vi "Get Part Information.vi"(8 "Error":errorcluster, 10 "station name":string, 11 "Part Type":string="WK") -> (0 "Error Out":errorcluster, 1 "Part Setup":T2={"Communication Type"=enum."None", "Send Messages to"=enum."Glass", "RAP Signal"=enum."None", "Motor Type"=enum."Smart Motor", "NVH Part Number"=0, "Turn Off Timer"=0, "Part Type"=""}, 2 "Switch Value Configuration":T7[](array[typedef]), 3 "Switch Configuration":T10[](array[typedef]), 4 "Motor Drift Compensation":i32[](array[numeric])=[25, 25, 25, 25, 25, 25, 25, 25], 5 "Seqence Info":T11[](array[typedef]), 6 "Hall Positions":i32[](array[numeric]), 7 "enable ps rem sense":bool, 9 "lvdt precision":T1)   [LabVIEW 2018]
uses:
  05.UserVI's/sequence/type defs/Sequence Info.ctl
  02.Type Def's/All Switch Configuration Cluster.ctl
  02.Type Def's/All Motions.ctl
  02.Type Def's/EOL Switch Value Configuration Cluster.ctl
  02.Type Def's/EOL Switch Max Min Check Cluster.ctl
  05.UserVI's/type defs/EOL Part Setup.ctl
  02.Type Def's/All Communication Types.ctl
  05.UserVI's/type defs/Communication with Motors.ctl
  05.UserVI's/type defs/RAP Signal Control.ctl
  05.UserVI's/type defs/EOL Motor Type.ctl
  05.UserVI's/LVDT's/lvdt precision.ctl
panel:
  # "Min"
  # "Max"
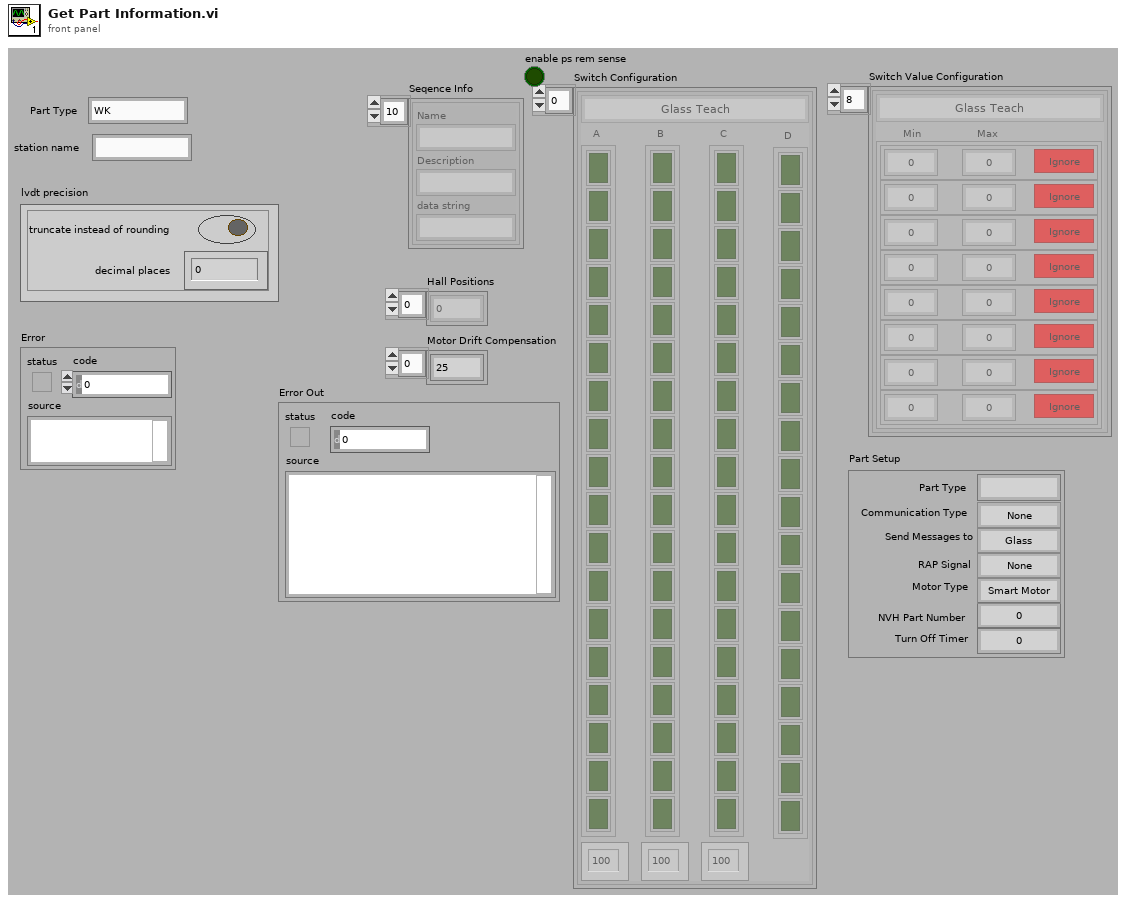
[diagram p1: front panel]
types:
  T1 = typedef "lvdt precision.ctl" = cluster{"truncate instead of rounding":bool, "decimal places":u8}
  T2 = typedef "EOL Part Setup.ctl" = cluster{"Communication Type":T3, "Send Messages to":T4, "RAP Signal":T5, "Motor Type":T6, "NVH Part Number":u16, "Turn Off Timer":u16, "Part Type":string}
  T3 = typedef "All Communication Types.ctl" = enum16{"None", "CAN", "RS 232", "RS 232 LIN", "GM LIN", "SnT LIN", "K Line", "Robel CAN", "P42M-Continental", "Inalfa SCU LIN", "Spare 3"}
  T4 = typedef "Communication with Motors.ctl" = enum16{"Glass", "Rollo", "Both"}
  T5 = typedef "RAP Signal Control.ctl" = enum16{"High", "Low", "None"}
  T6 = typedef "EOL Motor Type.ctl" = enum16{"Smart Motor", "Sensor Motor"}
  T7 = typedef "EOL Switch Value Configuration Cluster.ctl" = cluster{"All Motions":T8, "Array":T9[]}
  T8 = typedef "All Motions.ctl" = enum16{"Glass Teach", "Glass Slide Open", "Glass Slide Close", "Glass Vent Open", "Glass Vent Close", "Sunshade Teach", "Sunshade Open", "Sunshade Close", "Idle", "Sunshade Open 2", "Sunshade Close 2", "Glass Slide Open Sunshade Open", "Glass Slide Open Sunshade Close", "Glass Slide Close Sunshade Open", "Glass Slide Close Sunshade Close", "Glass Vent Open Sunshade Open", "Glass Vent Open Sunshade Close", "Glass Vent Close Sunshade Open", "Glass Vent Close Sunshade Close", "Express Glass Slide Open", "Express Glass Slide Close", "Express Glass Vent Open", "Express Glass Vent Close", "Express Sunshade Open", "Express Sunshade Close", "Express Sunshade Open 2", "Express Sunshade Close 2", "Express Glass Slide Open Sunshade Open", "Express Glass Slide Open Sunshade Close", "Express Glass Slide Close Sunshade Open", "Express Glass Slide Close Sunshade Close", "Express Glass Vent Open Sunshade Open", "Express Glass Vent Open Sunshade Close", "Express Glass Vent Close Sunshade Open", "Express Glass Vent Close Sunshade Close", "Goto Position Glass", "Goto Position Sunshade", "Sunshade Teach 2"}
  T9 = typedef "EOL Switch Max Min Check Cluster.ctl" = cluster{"Min":dbl, "Max":dbl, "Check?":bool}
  T10 = typedef "All Switch Configuration Cluster.ctl" = cluster{"All Motions":T8, "A":bool[], "B":bool[], "C":bool[], "D":bool[], "A activation time (ms)":u32, "B activation time (ms)":u32, "C activation time (ms)":u32}
  T11 = typedef "Sequence Info.ctl" = cluster{"Name":string, "Description":string, "data string":string}
  T12 = cluster{"Base Path":path, "Part Type":string, "station name":string, "Seqence Info":T11[], "Motion Switch Array":T10[], "Motion Switch Value Array":T7[], "Part Setup":T2, "Error":errorcluster, "Hall Positions":i32[], "Motor Drift Compensation":i32[], "enable ps rem sense":bool, "lvdt precision":T1, "hall parem name":string[]}
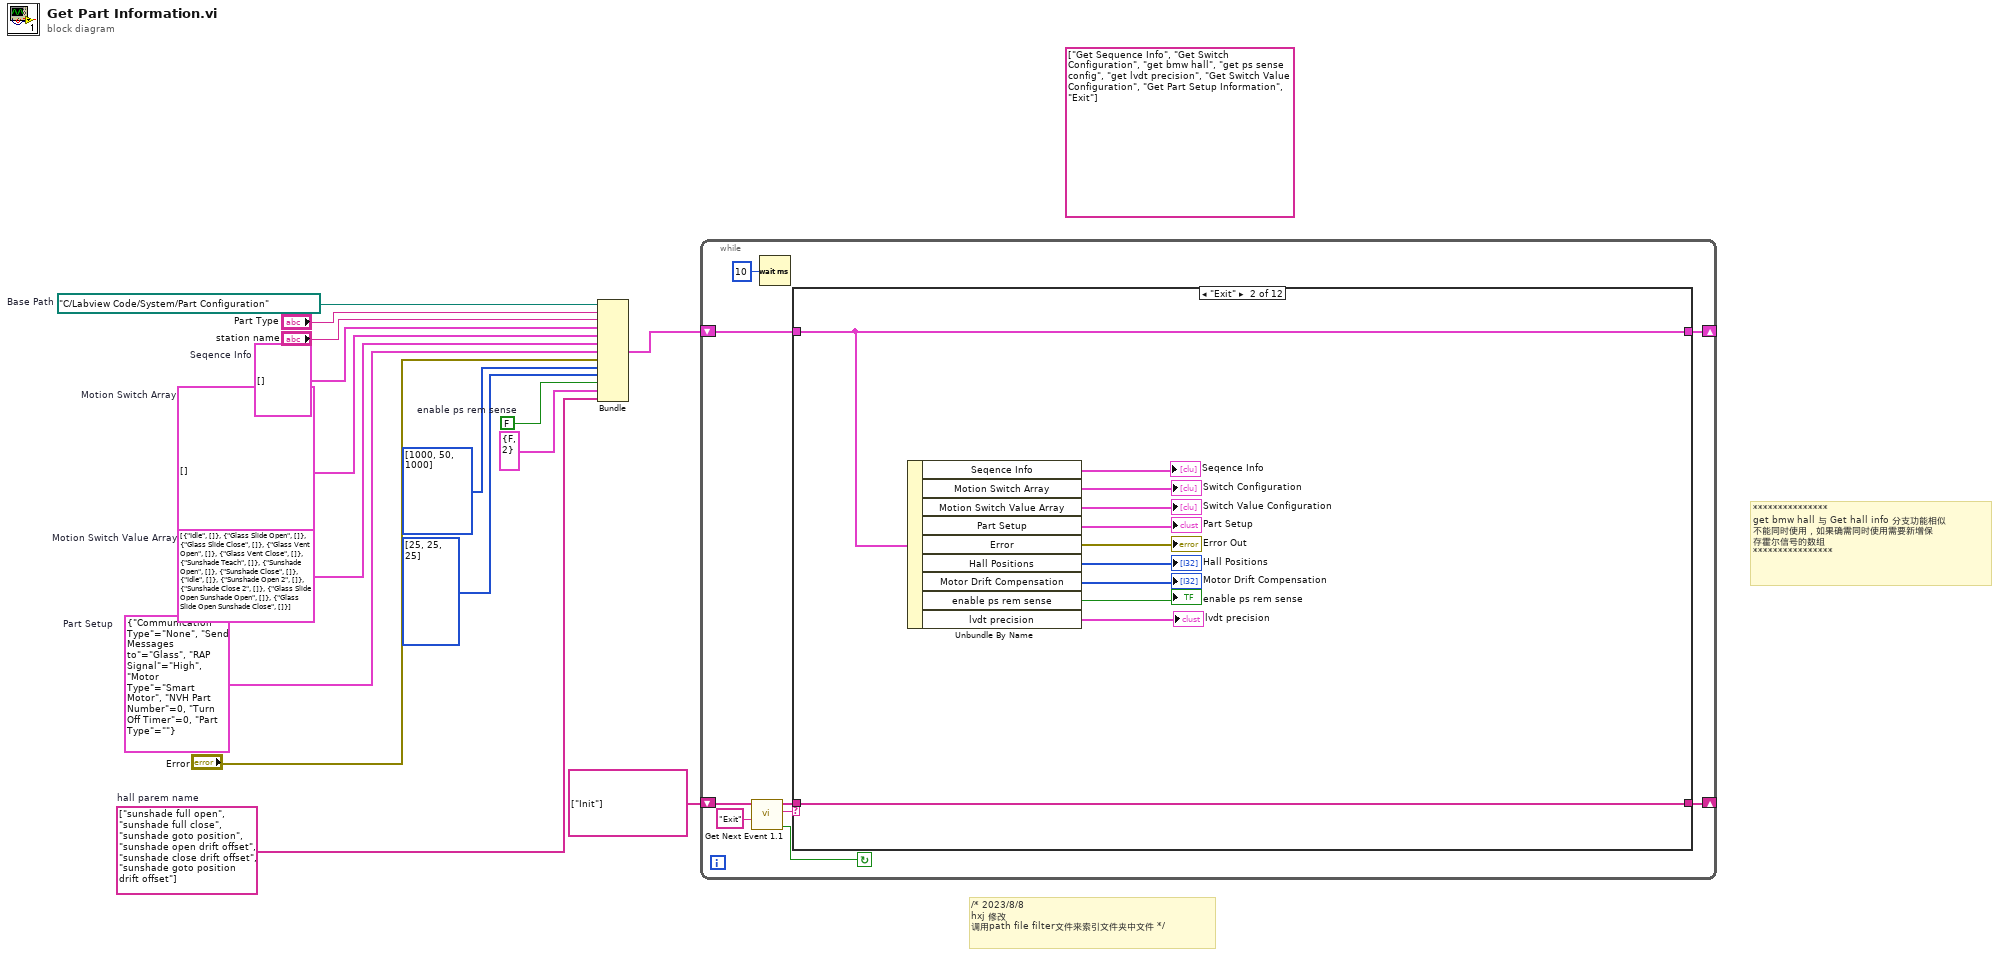
[diagram p0: block diagram]
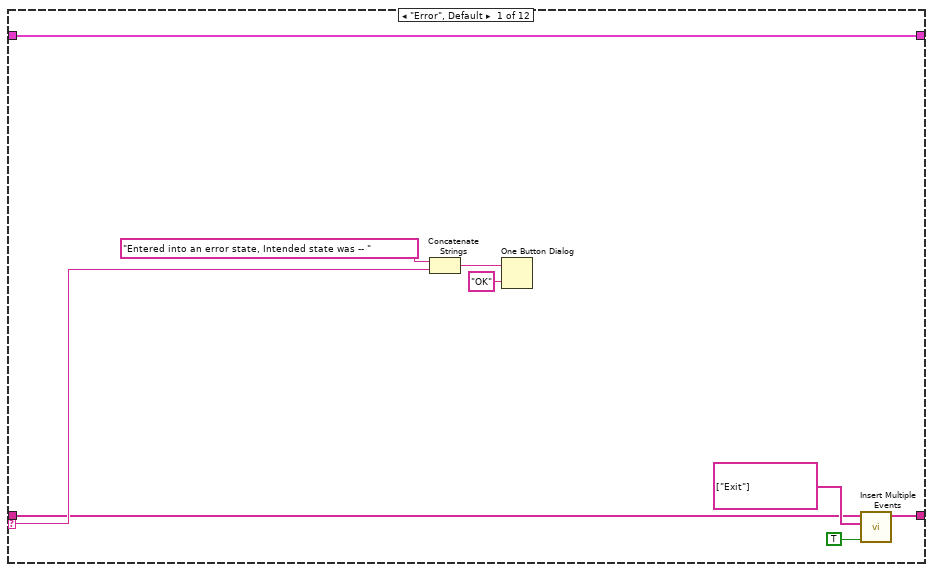
[diagram p2: hidden frame]
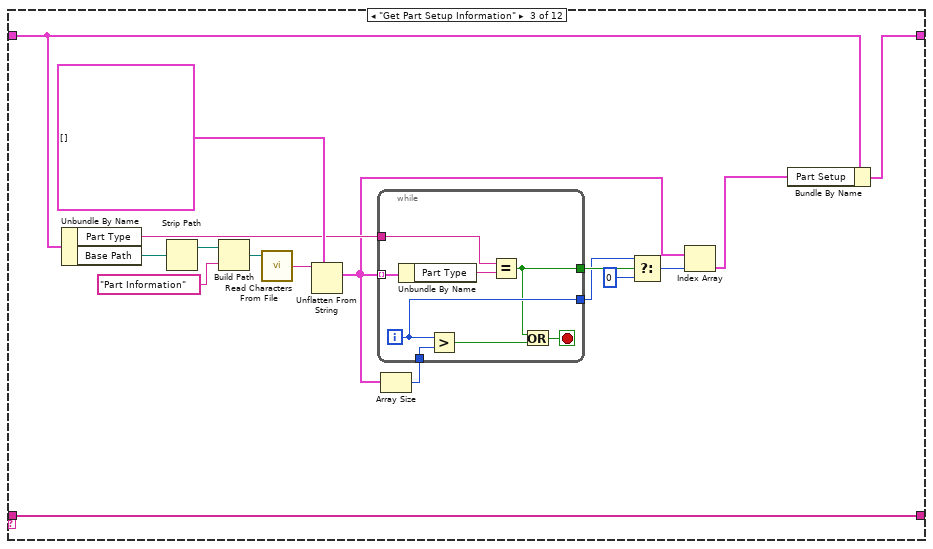
[diagram p3: hidden frame]
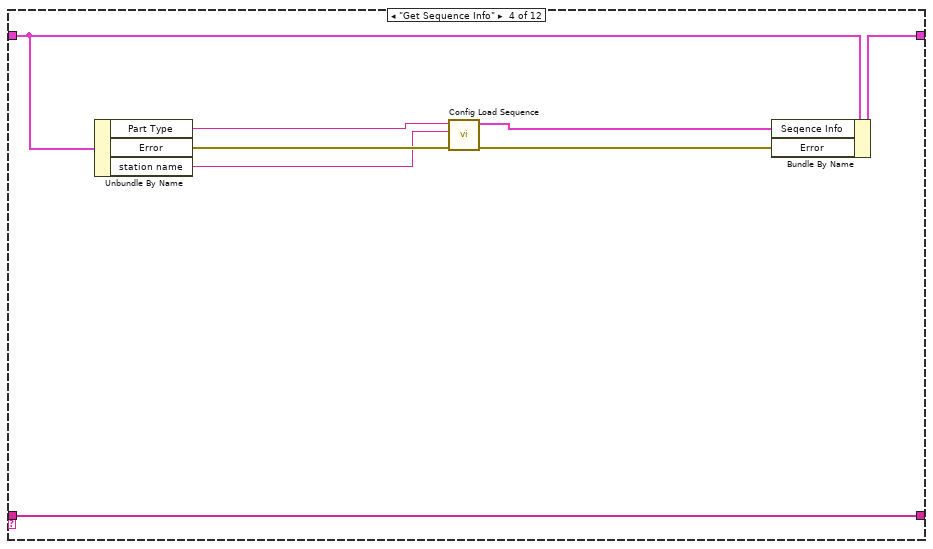
[diagram p4: hidden frame]
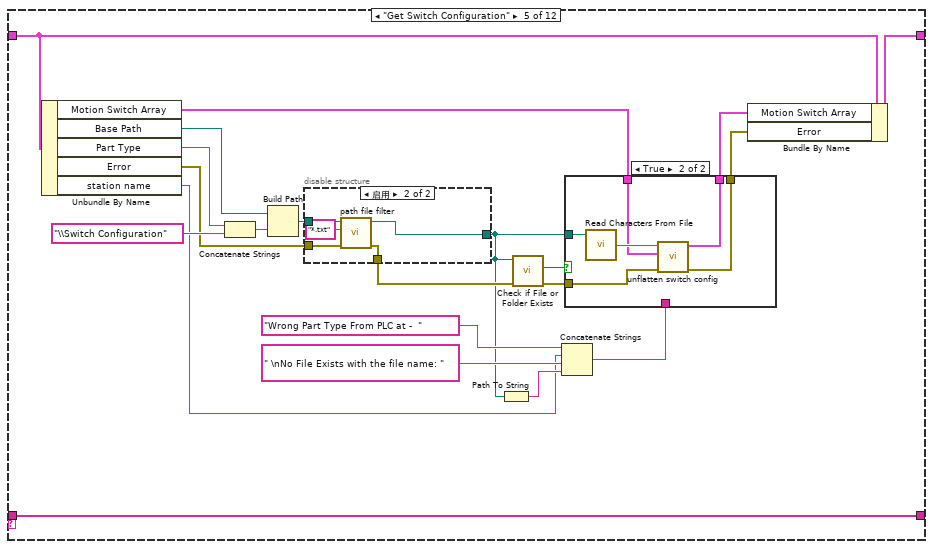
[diagram p5: hidden frame]
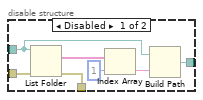
[diagram p6: hidden frame]
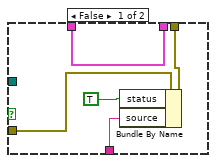
[diagram p7: hidden frame]
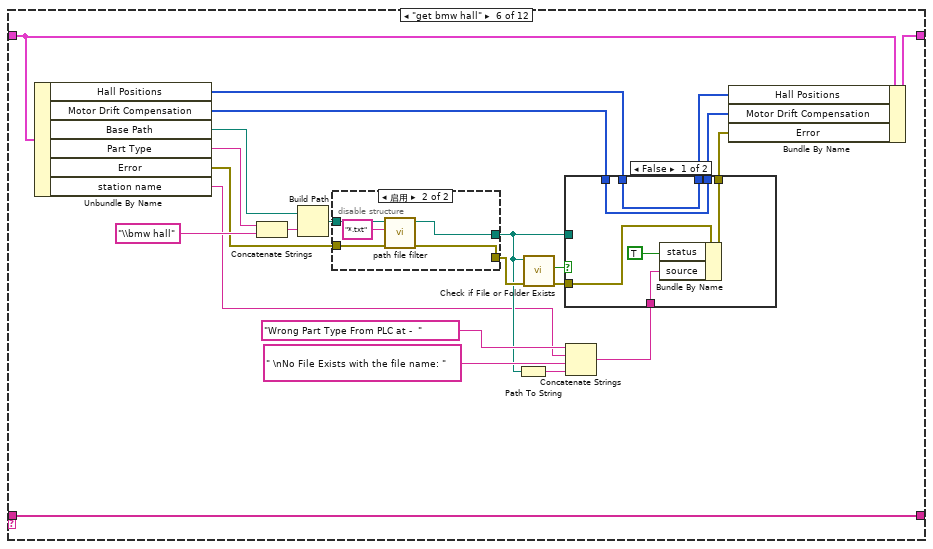
[diagram p8: hidden frame]
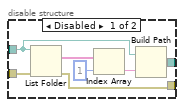
[diagram p9: hidden frame]
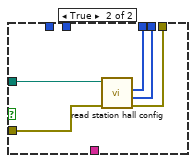
[diagram p10: hidden frame]
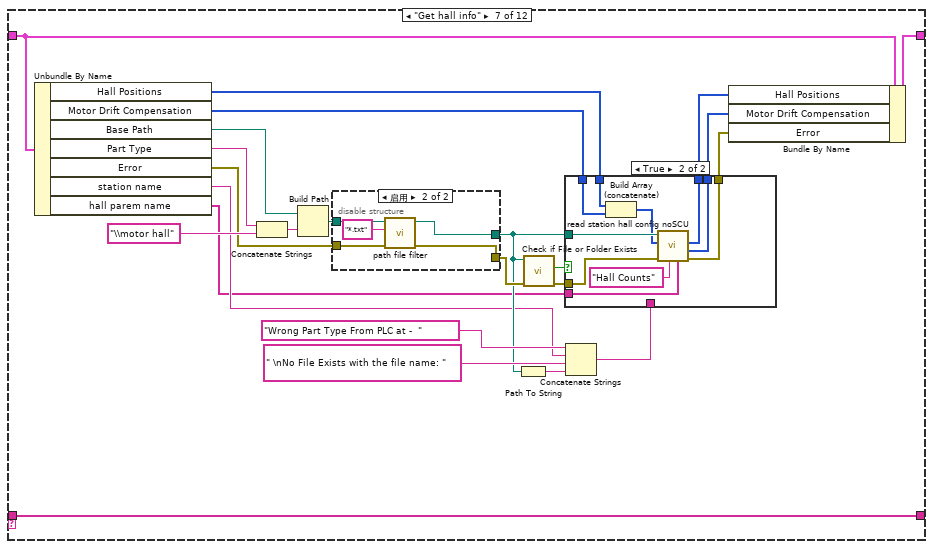
[diagram p11: hidden frame]
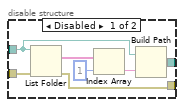
[diagram p12: hidden frame]
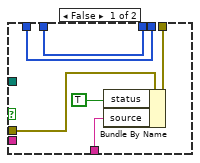
[diagram p13: hidden frame]
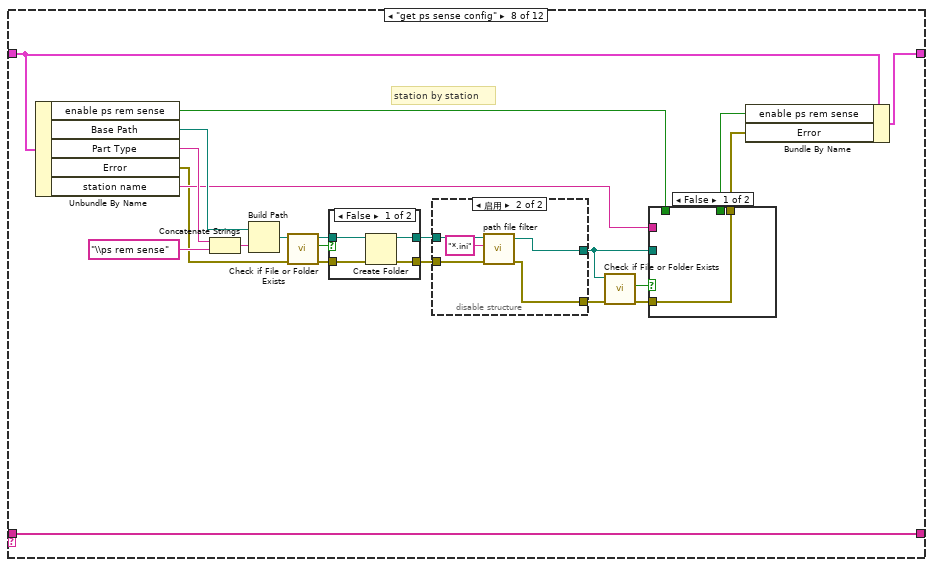
[diagram p14: hidden frame]
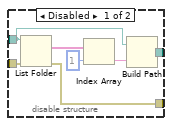
[diagram p15: hidden frame]
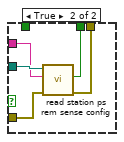
[diagram p17: hidden frame]
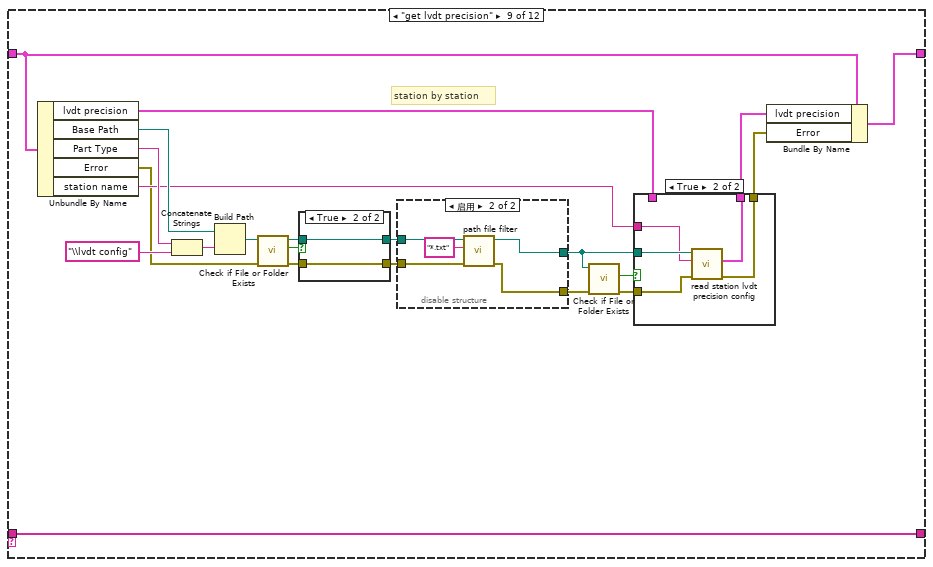
[diagram p18: hidden frame]
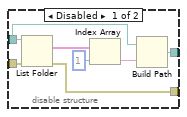
[diagram p19: hidden frame]
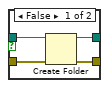
[diagram p20: hidden frame]
diagram:
  (unwired) string[] ["Get Sequence Info", "Get Switch Configuration", "get bmw hall", "get ps sense config", "get lvdt precision", "Get Switch Value Configuration", "Get Part Setup Information", "Exit"] ("event queue out")
  w1 = string[] ["sunshade full open", "sunshade full close", "sunshade goto position", "sunshade open drift offset", "sunshade close drift offset", "sunshade goto position drift offset"]  # hall parem name
  w3 = FALSE  # enable ps rem sense
  w6 = T2 {"Communication Type"=enum."None", "Send Messages to"=enum."Glass", "RAP Signal"=enum."High", "Motor Type"=enum."Smart Motor", "NVH Part Number"=0, "Turn Off Timer"=0, "Part Type"=""}  # Part Setup
  w9 = path "C:/Labview Code/System/Part Configuration"  # Base Path
  w11 = T7[] [{"All Motions"=enum."Idle", "Array"=[]}, {"All Motions"=enum."Glass Slide Open", "Array"=[]}, {"All Motions"=enum."Glass Slide Close", "Array"=[]}, {"All Motions"=enum."Glass Vent Open", "Array"=[]}, {"All Motions"=enum."Glass Vent Close", "Array"=[]}, {"All Motions"=enum."Sunshade Teach", "Array"=[]}, {"All Motions"=enum."Sunshade Open", "Array"=[]}, {"All Motions"=enum."Sunshade Close", "Array"=[]}, {"All Motions"=enum."Idle", "Array"=[]}, {"All Motions"=enum."Sunshade Open 2", "Array"=[]}, {"All Motions"=enum."Sunshade Close 2", "Array"=[]}, {"All Motions"=enum."Glass Slide Open Sunshade Open", "Array"=[]}, {"All Motions"=enum."Glass Slide Open Sunshade Close", "Array"=[]}]  # Motion Switch Value Array
  w12 = T10[] []  # Motion Switch Array
  w13 = T11[] []  # Seqence Info
  # "***************\nget bmw hall 与 Get hall info 分支功能相似\n不能同时使用，如果确需同时使用需要新增保\n存霍尔信号的数组 \n****************"
  # "/* 2023/8/8\nhxj 修改\n调用path file filter文件来索引文件夹中文件 */"
  n1 = Bundle("Base Path"=w9, "Part Type"="Part Type", "station name"="station name", "Seqence Info"=w13, "Motion Switch Array"=w12, "Motion Switch Value Array"=w11, "Part Setup"=w6, "Error"="Error", "Hall Positions"=i32[] [1000, 50, 1000], "Motor Drift Compensation"=i32[] [25, 25, 25], "enable ps rem sense"=w3, "lvdt precision"=T1 {"truncate instead of rounding"=FALSE, "decimal places"=2}, "hall parem name"=w1) -> (w15:T12)  [unwired: 1 in]
  n2 = while {
    shift-right: [w21] -> _
    shift-left: string[] ["Init"] ("event queue out") -> [w20]
    shift-right: [w16] -> _
    shift-left: w15 -> [w17]
    stop <- w24 continue-if-true
    n3 = call "Get Next Event 1.1.vi"("Exit Event"="Exit", "event queue in"=w20) -> ("Condition (Exit:F)"=w24:bool, "next event"=w23:string, "event queue out"=w22:string[])  [unwired: 6 in, 1 out]
    n4 = Wait (ms)(milliseconds to wait=u32 10) -> ()  [unwired: 1 out]
    n5 = case shown="\"Exit\"" w23 {
      selector: w23 -> [w31 _ _ _ _ _ _ _ _ _ _ _]
      tunnel: w22 -> [w25 w44 w61 w75 w91 w137 w184 w235 w281 w326 _ w363]
      tunnel: [w26 w44 w61 w75 w91 w137 w184 w235 w281 w326 w359 w364] -> w21
      tunnel: w17 -> [w33 w43 w60 w77 w95 w141 w188 w239 w285 w330 w358 w365]
      tunnel: [w33 w43 w59 w76 w92 w138 w185 w236 w282 w327 w358 w365] -> w16
      frame "Error", Default {
        n6 = Concatenate Strings("Entered into an error state, Intended state was -- " ("string"), w31) -> (w30:string)
        n7 = One Button Dialog(message=w30, button name ("OK")="OK") -> ()  [unwired: 1 out]
        n8 = call "Insert Multiple Events.vi"("Insert all? (T)"=TRUE, "Events to Insert"=string[] ["Exit"], "Event queue in"=w25) -> ("Event queue out"=w26:string[])  [unwired: 4 in]
      }
      frame "Exit" {
        n9 = Unbundle By Name(w43) -> ("Seqence Info"=→"Seqence Info":T11[], "Motion Switch Array"=→"Switch Configuration":T10[], "Motion Switch Value Array"=→"Switch Value Configuration":T7[], "Part Setup"=→"Part Setup":T2, "Error"=→"Error Out":errorcluster, "Hall Positions"=→"Hall Positions":i32[], "Motor Drift Compensation"=→"Motor Drift Compensation":i32[], "enable ps rem sense"=→"enable ps rem sense":bool, "lvdt precision"=→"lvdt precision":T1)
      }
      frame "Get Part Setup Information" {
        n10 = Unbundle By Name(w60) -> ("Part Type"=w56:string, "Base Path"=w46:path)
        n11 = Strip Path(path=w46) -> (stripped path=w48:path)  [unwired: 1 out]
        n12 = Build Path(base path=w48, name or relative path="Part Information") -> (appended path=w45:path)
        n13 = call <vilib>:"Read Characters From File.vi"("file path (dialog if empty)"=w45) -> ("character string"=w58:string)  [unwired: 5 in, 3 out]
        n14 = Unflatten From String(type=T2[] [] ("Array"), binary string=w58) -> (value=w50:T2[])  [unwired: 3 in, 2 out]
        n15 = Array Size(array=w50) -> (size(s)=w55:i32)
        n16 = while {
          tunnel: w50 -> [w69] mode=indexing
          tunnel: w56 -> [w67]
          tunnel: w55 -> [w66]
          tunnel: [w63] -> w53
          tunnel: [w62] -> w54
          i -> [w63]
          stop <- w65 stop-if-true
          n17 = Unbundle By Name(w69) -> ("Part Type"=w68:string)
          n18 = Greater?(x=w63, y=w66) -> (0:w64:bool)
          n19 = Equal?(x=w67, y=w68) -> (x = y?=w62:bool)
          n20 = Or(x=w62, y=w64) -> (x .or. y?=w65:bool)
        }
        n21 = Select(t=w53, s=w54, f=0) -> (s? t:f=w51:i32)
        n22 = Index Array(array=w50, index=w51) -> (element=w49:T2)
        n23 = Bundle By Name(cluster=w60, "Part Setup"=w49) -> (w59:T12)
      }
      frame "Get Sequence Info" {
        n24 = Unbundle By Name(w77) -> ("Part Type"=w71:string, "Error"=w72:errorcluster, "station name"=w70:string)
        n25 = call "Config Load Sequence.vi"("Sys Error In"=w72, "Station"=w70, "Part Type"=w71) -> ("Sys Error Out"=w73:errorcluster, "Seqence Info"=w74:T11[])  [unwired: 4 in, 3 out]
        n26 = Bundle By Name(cluster=w77, "Seqence Info"=w74, "Error"=w73) -> (w76:T12)
      }
      frame "Get Switch Configuration" {
        n27 = Unbundle By Name(w95) -> ("Motion Switch Array"=w89:T10[], "Base Path"=w94:path, "Part Type"=w93:string, "Error"=w84:errorcluster, "station name"=w78:string)
        n28 = Concatenate Strings(w93, "\\Switch Configuration" ("string")) -> (w96:string)
        n29 = Build Path(base path=w94, name or relative path=w96) -> (appended path=w98:path)
        n30 = disable-structure shown="启用" {
          disable-tunnel: w98 -> [w103 w110]
          disable-tunnel: [w102 w108] -> w86
          disable-tunnel: w84 -> [w101 w109]
          disable-tunnel: [w100 w106] -> w80
          frame Disabled {
            n31 = List Folder(path=w103, error in=w101) -> (filenames=w104:string[], error out=w102:errorcluster)  [unwired: 2 in, 2 out]
            n32 = Index Array(array=w104, index=1 ("索引")) -> (element=w105:string)
            n33 = Build Path(base path=w103, name or relative path=w105) -> (appended path=w100:path)
          }
          frame Enabled {
            n34 = call "path file filter.vi"("Sys Error In"=w109, "file type"="*.txt", "path"=w110) -> ("错误输出"=w108:errorcluster, "File path"=w106:path)  [unwired: 7 in]
          }
        }
        n35 = Path To String(path=w80) -> (string=w83:string)
        n36 = call <vilib>:"Check if File or Folder Exists.vi"("error in (no error)"=w86, "path"=w80) -> ("error out"=w85:errorcluster, "file or folder exists?"=w90:bool)  [unwired: 7 in, 1 out]
        n37 = Concatenate Strings("Wrong Part Type From PLC at -  " ("string"), w78, " \nNo File Exists with the file name: " ("string"), w83) -> (w79:string)
        n38 = case shown="True" w90 {
          tunnel: w89 -> [w115 w119]
          tunnel: [w115 w118] -> w88
          tunnel: [w114 w116] -> w87
          tunnel: w80 -> [_ w121]
          tunnel: w79 -> [w112 _]
          tunnel: w85 -> [w111 w117]
          frame False {
            n39 = Bundle By Name(cluster=w111, "status"=TRUE, "source"=w112) -> (w114:errorcluster)
          }
          frame True {
            n40 = call <vilib>:"Read Characters From File.vi"("file path (dialog if empty)"=w121) -> ("character string"=w120:string)  [unwired: 5 in, 3 out]
            n41 = call "unflatten switch config.vi"("error in (no error)"=w117, "Motion Switch Array in"=w119, "string"=w120) -> ("error out"=w116:errorcluster, "Motion Switch Array out"=w118:T10[])  [unwired: 7 in]
          }
        }
        n42 = Bundle By Name(cluster=w95, "Motion Switch Array"=w88, "Error"=w87) -> (w92:T12)
      }
      frame "get bmw hall" {
        n43 = Unbundle By Name(w141) -> ("Hall Positions"=w124:i32[], "Motor Drift Compensation"=w123:i32[], "Base Path"=w140:path, "Part Type"=w139:string, "Error"=w122:errorcluster, "station name"=w126:string)
        n44 = Concatenate Strings(w139, "\\bmw hall" ("string")) -> (w142:string)
        n45 = Build Path(base path=w140, name or relative path=w142) -> (appended path=w144:path)
        n46 = disable-structure shown="启用" {
          disable-tunnel: w144 -> [w149 w156]
          disable-tunnel: [w145 w155] -> w133
          disable-tunnel: [w148 w153] -> w128
          disable-tunnel: w122 -> [w146 w154]
          frame Disabled {
            n47 = List Folder(path=w149, error in=w146) -> (filenames=w150:string[], error out=w145:errorcluster)  [unwired: 2 in, 2 out]
            n48 = Index Array(array=w150, index=1 ("索引")) -> (element=w151:string)
            n49 = Build Path(base path=w149, name or relative path=w151) -> (appended path=w148:path)
          }
          frame Enabled {
            n50 = call "path file filter.vi"("Sys Error In"=w154, "file type"="*.txt", "path"=w156) -> ("错误输出"=w155:errorcluster, "File path"=w153:path)  [unwired: 7 in]
          }
        }
        n51 = Path To String(path=w128) -> (string=w131:string)
        n52 = call <vilib>:"Check if File or Folder Exists.vi"("error in (no error)"=w133, "path"=w128) -> ("error out"=w132:errorcluster, "file or folder exists?"=w136:bool)  [unwired: 7 in, 1 out]
        n53 = Concatenate Strings("Wrong Part Type From PLC at -  " ("string"), w126, " \nNo File Exists with the file name: " ("string"), w131) -> (w127:string)
        n54 = case shown="False" w136 {
          tunnel: [w157 w166] -> w135
          tunnel: [w162 w164] -> w134
          tunnel: w128 -> [_ w167]
          tunnel: w127 -> [w160 _]
          tunnel: w132 -> [w159 w165]
          tunnel: [w158 w163] -> w125
          tunnel: w124 -> [w158 _]
          tunnel: w123 -> [w157 _]
          frame False {
            n55 = Bundle By Name(cluster=w159, "status"=TRUE, "source"=w160) -> (w162:errorcluster)
          }
          frame True {
            n56 = call "read station hall config.vi"("error in"=w165, "configuration file path in"=w167) -> ("error out"=w164:errorcluster, "Motor Drift Compensation"=w166:i32[], "Hall Positions"=w163:i32[])  [unwired: 6 in, 1 out]
          }
        }
        n57 = Bundle By Name(cluster=w141, "Hall Positions"=w125, "Motor Drift Compensation"=w135, "Error"=w134) -> (w138:T12)
      }
      frame "Get hall info" {
        n58 = Unbundle By Name(w188) -> ("Hall Positions"=w171:i32[], "Motor Drift Compensation"=w170:i32[], "Base Path"=w187:path, "Part Type"=w186:string, "Error"=w169:errorcluster, "station name"=w173:string, "hall parem name"=w168:string[])
        n59 = Concatenate Strings(w186, "\\motor hall" ("string")) -> (w189:string)
        n60 = Build Path(base path=w187, name or relative path=w189) -> (appended path=w191:path)
        n61 = disable-structure shown="启用" {
          disable-tunnel: w191 -> [w196 w203]
          disable-tunnel: [w192 w202] -> w180
          disable-tunnel: [w195 w200] -> w175
          disable-tunnel: w169 -> [w193 w201]
          frame Disabled {
            n62 = List Folder(path=w196, error in=w193) -> (filenames=w197:string[], error out=w192:errorcluster)  [unwired: 2 in, 2 out]
            n63 = Index Array(array=w197, index=1 ("索引")) -> (element=w198:string)
            n64 = Build Path(base path=w196, name or relative path=w198) -> (appended path=w195:path)
          }
          frame Enabled {
            n65 = call "path file filter.vi"("Sys Error In"=w201, "file type"="*.txt", "path"=w203) -> ("错误输出"=w202:errorcluster, "File path"=w200:path)  [unwired: 7 in]
          }
        }
        n66 = Path To String(path=w175) -> (string=w178:string)
        n67 = call <vilib>:"Check if File or Folder Exists.vi"("error in (no error)"=w180, "path"=w175) -> ("error out"=w179:errorcluster, "file or folder exists?"=w183:bool)  [unwired: 7 in, 1 out]
        n68 = Concatenate Strings("Wrong Part Type From PLC at -  " ("string"), w173, " \nNo File Exists with the file name: " ("string"), w178) -> (w174:string)
        n69 = case shown="True" w183 {
          tunnel: [w204 w218] -> w182
          tunnel: [w209 w216] -> w181
          tunnel: w175 -> [_ w219]
          tunnel: w174 -> [w207 _]
          tunnel: w179 -> [w206 w217]
          tunnel: [w205 w215] -> w172
          tunnel: w171 -> [w205 w212]
          tunnel: w170 -> [w204 w211]
          tunnel: w168 -> [_ w214]
          frame False {
            n70 = Bundle By Name(cluster=w206, "status"=TRUE, "source"=w207) -> (w209:errorcluster)
          }
          frame True {
            n71 = Build Array (concatenate)(w212, w211) -> (w210:i32[])
            n72 = call "read station hall config noSCU.vi"("name"=w214, "section"="Hall Counts", "error in"=w217, "default value"=w210, "configuration file path in"=w219) -> ("error out"=w216:errorcluster, "Motor Drift Compensation"=w218:i32[], "Hall Positions"=w215:i32[])  [unwired: 3 in, 1 out]
          }
        }
        n73 = Bundle By Name(cluster=w188, "Hall Positions"=w172, "Motor Drift Compensation"=w182, "Error"=w181) -> (w185:T12)
      }
      frame "get ps sense config" {
        # "station by station"
        n74 = Unbundle By Name(w239) -> ("enable ps rem sense"=w228:bool, "Base Path"=w238:path, "Part Type"=w237:string, "Error"=w226:errorcluster, "station name"=w227:string)
        n75 = Concatenate Strings(w237, "\\ps rem sense" ("string")) -> (w240:string)
        n76 = Build Path(base path=w238, name or relative path=w240) -> (appended path=w224:path)
        n77 = call <vilib>:"Check if File or Folder Exists.vi"("error in (no error)"=w226, "path"=w224) -> ("error out"=w220:errorcluster, "file or folder exists?"=w225:bool, "dup path"=w222:path)  [unwired: 7 in]
        n78 = case shown="False" w225 {
          tunnel: [w255 w259] -> w223
          tunnel: w222 -> [w257 w259]
          tunnel: [w254 w258] -> w221
          tunnel: w220 -> [w256 w258]
          frame False {
            n79 = Create Folder(path (use dialog)=w257, error in=w256) -> (created path=w255:path, error out=w254:errorcluster)  [unwired: 1 in, 1 out]
          }
          frame True {
          }
        }
        n80 = disable-structure shown="启用" {
          disable-tunnel: [w246 w250] -> w232
          disable-tunnel: [w245 w251] -> w230
          disable-tunnel: w223 -> [w244 w253]
          disable-tunnel: w221 -> [w243 w252]
          frame Disabled {
            n81 = List Folder(path=w244, error in=w243) -> (filenames=w247:string[], error out=w246:errorcluster)  [unwired: 2 in, 2 out]
            n82 = Index Array(array=w247, index=1 ("索引")) -> (element=w248:string)
            n83 = Build Path(base path=w244, name or relative path=w248) -> (appended path=w245:path)
          }
          frame Enabled {
            n84 = call "path file filter.vi"("Sys Error In"=w252, "file type"="*.ini", "path"=w253) -> ("错误输出"=w250:errorcluster, "File path"=w251:path)  [unwired: 7 in]
          }
        }
        n85 = call <vilib>:"Check if File or Folder Exists.vi"("error in (no error)"=w232, "path"=w230) -> ("error out"=w231:errorcluster, "file or folder exists?"=w234:bool)  [unwired: 7 in, 1 out]
        n86 = case shown="False" w234 {
          tunnel: [w260 w263] -> w233
          tunnel: w230 -> [_ w265]
          tunnel: w231 -> [w260 w264]
          tunnel: [_ w261] -> w229
          tunnel: w228 -> [_ _]
          tunnel: w227 -> [_ w262]
          frame False {
          }
          frame True {
            n87 = call "read station ps rem sense config.vi"("error in"=w264, "station"=w262, "configuration file path in"=w265) -> ("error out"=w263:errorcluster, "enable remote sense"=w261:bool)  [unwired: 6 in, 1 out]
          }
        }
        n88 = Bundle By Name(cluster=w239, "enable ps rem sense"=w229, "Error"=w233) -> (w236:T12)
      }
      frame "get lvdt precision" {
        # "station by station"
        n89 = Unbundle By Name(w285) -> ("lvdt precision"=w274:T1, "Base Path"=w284:path, "Part Type"=w283:string, "Error"=w272:errorcluster, "station name"=w273:string)
        n90 = Concatenate Strings(w283, "\\lvdt config" ("string")) -> (w286:string)
        n91 = Build Path(base path=w284, name or relative path=w286) -> (appended path=w270:path)
        n92 = call <vilib>:"Check if File or Folder Exists.vi"("error in (no error)"=w272, "path"=w270) -> ("error out"=w267:errorcluster, "file or folder exists?"=w271:bool, "dup path"=w269:path)  [unwired: 7 in]
        n93 = case shown="True" w271 {
          tunnel: [w301 w305] -> w266
          tunnel: w269 -> [w303 w305]
          tunnel: [w300 w304] -> w268
          tunnel: w267 -> [w302 w304]
          frame False {
            n94 = Create Folder(path (use dialog)=w303, error in=w302) -> (created path=w301:path, error out=w300:errorcluster)  [unwired: 1 in, 1 out]
          }
          frame True {
          }
        }
        n95 = disable-structure shown="启用" {
          disable-tunnel: [w292 w297] -> w278
          disable-tunnel: [w291 w296] -> w276
          disable-tunnel: w268 -> [w290 w298]
          disable-tunnel: w266 -> [w288 w299]
          frame Disabled {
            n96 = List Folder(path=w288, error in=w290) -> (filenames=w293:string[], error out=w292:errorcluster)  [unwired: 2 in, 2 out]
            n97 = Index Array(array=w293, index=1 ("索引")) -> (element=w294:string)
            n98 = Build Path(base path=w288, name or relative path=w294) -> (appended path=w291:path)
          }
          frame Enabled {
            n99 = call "path file filter.vi"("Sys Error In"=w298, "file type"="*.txt", "path"=w299) -> ("错误输出"=w297:errorcluster, "File path"=w296:path)  [unwired: 7 in]
          }
        }
        n100 = call <vilib>:"Check if File or Folder Exists.vi"("error in (no error)"=w278, "path"=w276) -> ("error out"=w277:errorcluster, "file or folder exists?"=w280:bool)  [unwired: 7 in, 1 out]
        n101 = case shown="True" w280 {
          tunnel: [w307 w310] -> w279
          tunnel: w276 -> [_ w312]
          tunnel: w277 -> [w307 w311]
          tunnel: [w306 w308] -> w275
          tunnel: w274 -> [w306 _]
          tunnel: w273 -> [_ w309]
          frame False {
          }
          frame True {
            n102 = call "read station lvdt precision config.vi"("error in"=w311, "station"=w309, "configuration file path in"=w312) -> ("error out"=w310:errorcluster, "lvdt precision"=w308:T1)  [unwired: 6 in, 1 out]
          }
        }
        n103 = Bundle By Name(cluster=w285, "lvdt precision"=w275, "Error"=w279) -> (w282:T12)
      }
      frame "Get Switch Value Configuration" {
        n104 = Unbundle By Name(w330) -> ("Motion Switch Value Array"=w324:T7[], "Base Path"=w329:path, "Part Type"=w328:string, "Error"=w321:errorcluster, "station name"=w313:string)
        n105 = Concatenate Strings(w328, "\\Switch Value Configuration" ("string")) -> (w331:string)
        n106 = Build Path(base path=w329, name or relative path=w331) -> (appended path=w333:path)
        n107 = disable-structure shown="启用" {
          disable-tunnel: w333 -> [w338 w345]
          disable-tunnel: w321 -> [w337 w344]
          disable-tunnel: [w336 w343] -> w320
          disable-tunnel: [w335 w342] -> w315
          frame Disabled {
            n108 = List Folder(path=w338, error in=w337) -> (filenames=w339:string[], error out=w336:errorcluster)  [unwired: 2 in, 2 out]
            n109 = Index Array(array=w339, index=1 ("索引")) -> (element=w340:string)
            n110 = Build Path(base path=w338, name or relative path=w340) -> (appended path=w335:path)
          }
          frame Enabled {
            n111 = call "path file filter.vi"("Sys Error In"=w344, "file type"="*.txt", "path"=w345) -> ("错误输出"=w343:errorcluster, "File path"=w342:path)  [unwired: 7 in]
          }
        }
        n112 = Path To String(path=w315) -> (string=w318:string)
        n113 = call <vilib>:"Check if File or Folder Exists.vi"("error in (no error)"=w320, "path"=w315) -> ("error out"=w319:errorcluster, "file or folder exists?"=w325:bool)  [unwired: 7 in, 1 out]
        n114 = Concatenate Strings("Wrong Part Type From PLC at -  " ("string"), w313, " \nNo File Exists with the file name: " ("string"), w318) -> (w314:string)
        n115 = case shown="True" w325 {
          tunnel: w324 -> [w350 w355]
          tunnel: [w350 w354] -> w323
          tunnel: [w349 w353] -> w322
          tunnel: w315 -> [_ w352]
          tunnel: w314 -> [w347 _]
          tunnel: w319 -> [w346 w351]
          frame False {
            n116 = Bundle By Name(cluster=w346, "status"=TRUE, "source"=w347) -> (w349:errorcluster)
          }
          frame True {
            n117 = call <vilib>:"Read Characters From File.vi"("file path (dialog if empty)"=w352) -> ("character string"=w356:string)  [unwired: 5 in, 3 out]
            n118 = Unflatten From String(type=w355, binary string=w356, error in (no error)=w351) -> (value=w354:T7[], error out=w353:errorcluster)  [unwired: 2 in, 1 out]
          }
        }
        n119 = Bundle By Name(cluster=w330, "Motion Switch Value Array"=w323, "Error"=w322) -> (w327:T12)
      }
      frame "Init" {
        # "/* 2023/7/18\nhxj  修改\n新增选择分支，根据产线需求获取初始化信息 */"
        n120 = Unbundle By Name(w358) -> ("Part Type"=w357:string)
        n121 = case shown="Default" w357 {
          tunnel: [string[] ["Get Sequence Info", "Get Switch Configuration", "Get Switch Value Configuration", "Get Part Setup Information", "Exit"] ("event queue out")] -> w359
          frame Default {
          }
        }
      }
      frame "New State" {
        n122 = call "Insert Multiple Events.vi"("Insert all? (T)"=TRUE, "Events to Insert"=string[] [], "Event queue in"=w363) -> ("Event queue out"=w364:string[])  [unwired: 4 in]
      }
    }
  }
